vi "MultiModuleAssembly.vi"() -> ()   [LabVIEW 2019]
panel:
  in  "GoHome":bool
  out "Error Out":errorcluster
  in  "Error In":errorcluster
  out "CurrentGlueCommand":string
  in  "GlPatternPCB2":path=path "C:/Users/TTUHEP/Documents/LabVIEW/Data/Patterns/NSH_10-28-2021_rotated1_Minus120degrees_edgesModified_circlesFirst_Combined_version2.ngc"
  in  "Position2":bool=TRUE
  in  "Position1":bool=TRUE
  in  "Glue2":bool=TRUE
  in  "Glue1":bool=TRUE
  in  "Operations2":T1={"GoToToolPos"=TRUE, "PickTool"=TRUE, "GoToSenPCB"=TRUE, "PickSiPCB"=TRUE, "GoToBP"=TRUE, "DropTool"=TRUE}
  in  "Zone":enum16{"ZoneA", "ZoneB", "ZoneC", "ZoneD"}(ring)
  in  "AssmbType":enum16{"Sensor", "PCB"}(ring)=enum."PCB"
  in  "Operations1":T1={"GoToToolPos"=TRUE, "PickTool"=TRUE, "GoToSenPCB"=TRUE, "PickSiPCB"=TRUE, "GoToBP"=TRUE, "DropTool"=TRUE}
  in  "PressureSiPCB2":dbl[](array[numeric])=[15.0, 14.0, 8.0, 0.0]
  in  "PressureBPSi2":dbl[](array[numeric])=[30.0, 30.0, 15.0, 0.0]
  in  "SyringePosition2":T2={"SyringeX"=385.441, "SyringeY"=892.714, "SyringeZ"=75.0} {"SyringeX" format="%#_13g"; "SyringeY" format="%#_13g"}
  in  "SyringePosition1":T2={"SyringeX"=333.933, "SyringeY"=1082.586, "SyringeZ"=74.0} {"SyringeX" format="%#_13g"; "SyringeY" format="%#_13g"}
  in  "PressureSiPCB1":dbl[](array[numeric])=[15.0, 14.0, 8.0, 0.0]
  in  "PressureBPSi1":dbl[](array[numeric])=[30.0, 30.0, 15.0, 0.0]
  in  "GlueVISA":refnum<visa-resource-name>="COM5"
  in  "GlPatternSi":path=path "C:/Users/TTUHEP/Documents/LabVIEW/Data/Patterns/Final_Patern/PCB_base_10-25-2021_3layers_Combined_Final.ngc"
  in  "GlPatternPCB1":path=path "C:/Users/TTUHEP/Documents/LabVIEW/Data/Patterns/NSH_10-28-2021_rotated1_Minus120degrees_edgesModified_circlesFirst_Combined_version2.ngc"
  in  "SyringeToPlateGap(um)":string="330"
  in  "Initialize":T3
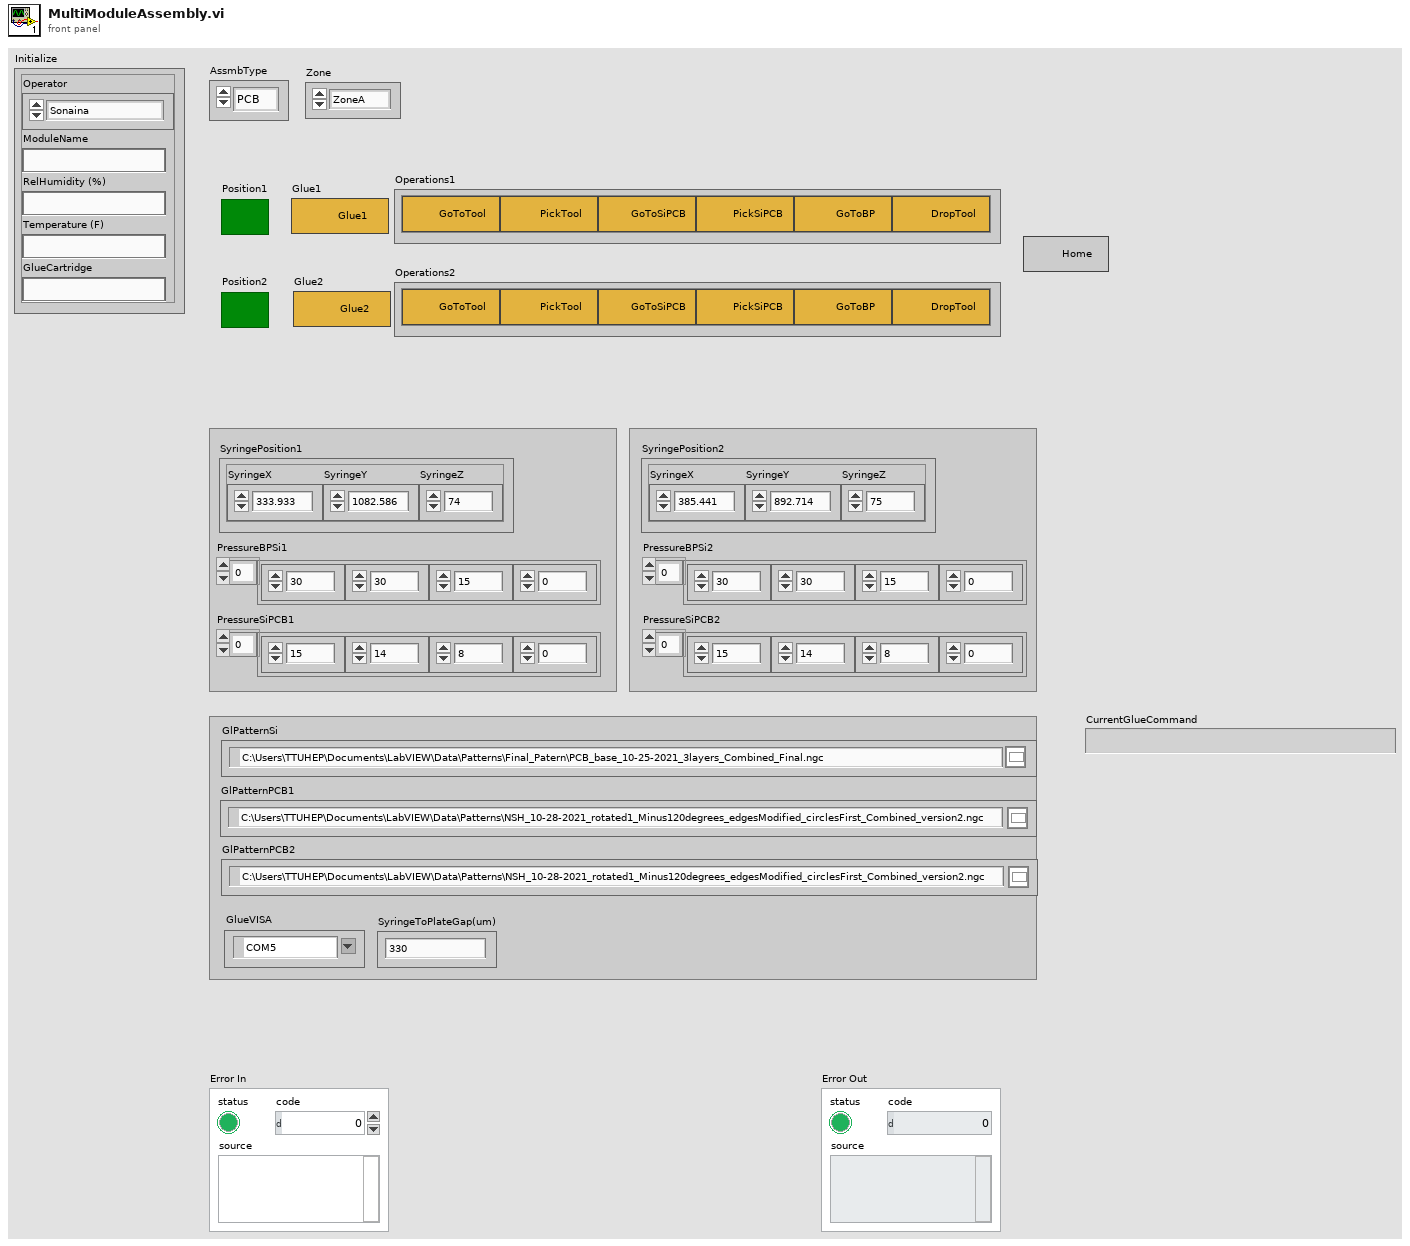
[diagram p1: front panel]
types:
  T1 = cluster{"GoToToolPos":bool, "PickTool":bool, "GoToSenPCB":bool, "PickSiPCB":bool, "GoToBP":bool, "DropTool":bool}
  T2 = cluster{"SyringeX":dbl, "SyringeY":dbl, "SyringeZ":dbl}
  T3 = cluster{"Operator":enum16{"Sonaina", "Vladimir", "Vinay", "Other"}, "ModuleName":string, "RelHumidity (%)":string, "Temperature (F)":string, "GlueCartridge":string}
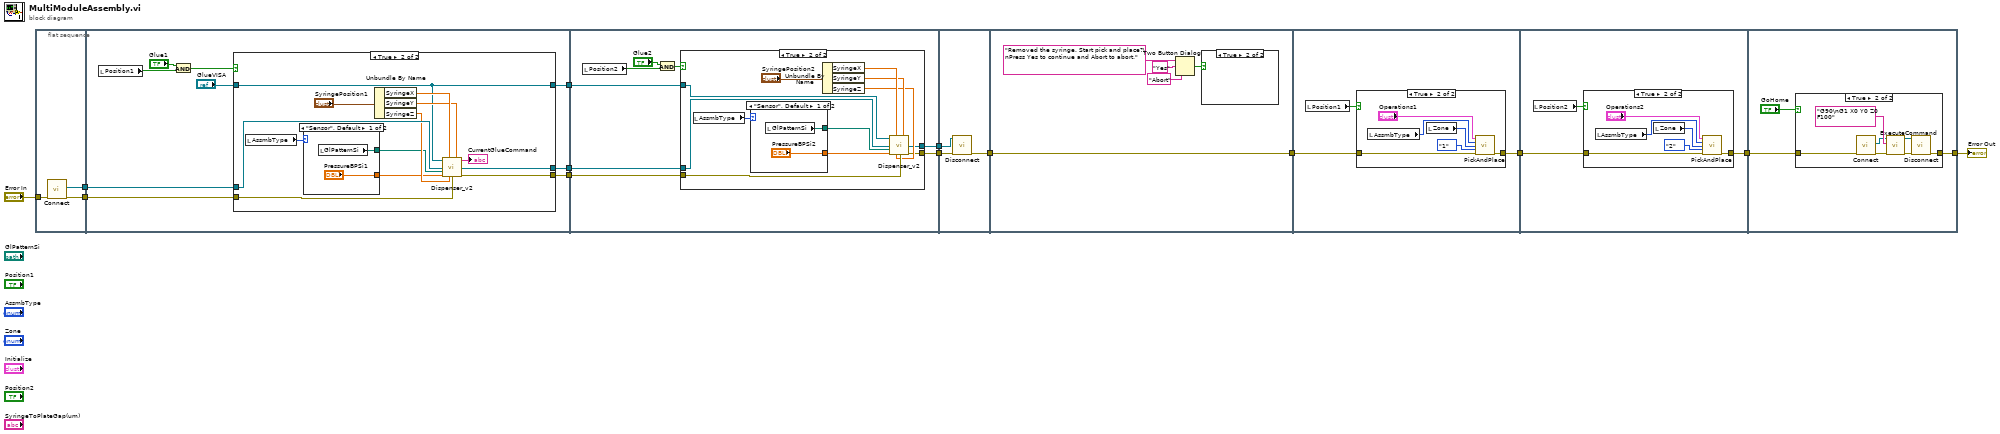
[diagram p0: block diagram]
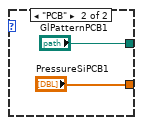
[diagram p3: hidden frame]
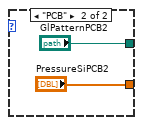
[diagram p5: hidden frame]
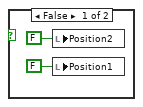
[diagram p6: hidden frame]
diagram:
  n1 = flat-sequence {
    tunnel: [w16] -> w13
    tunnel: [w15] -> w12
    tunnel: "Error In" -> [w14]
    tunnel: w13 -> [w25]
    tunnel: w12 -> [w24]
    tunnel: [w20] -> w11
    tunnel: [w19] -> w10
    tunnel: [w17] -> w7
    tunnel: w11 -> [w50]
    tunnel: w10 -> [w49]
    tunnel: [w48] -> w9
    tunnel: [w47] -> w8
    tunnel: w7 -> [w46]
    tunnel: w9 -> [w74]
    tunnel: w8 -> [w73]
    tunnel: [w72] -> w2
    tunnel: w2 -> [w79]
    tunnel: [w79] -> w1
    tunnel: w1 -> [w84]
    tunnel: [w82] -> w6
    tunnel: w6 -> [w93]
    tunnel: [w92] -> w3
    tunnel: [w103] -> w4
    tunnel: w3 -> [w102]
    frame #0 {
      n2 = call "Connect.vi"("error in (no error)"=w14) -> ("error out"=w15:errorcluster, "controller"=w16:refnum<k24>)  [unwired: 9 in]
    }
    frame #1 {
      n3 = local read "Position1"() -> (w22:bool)
      n4 = And(x="Glue1", y=w22) -> (x .and. y?=w21:bool)
      n5 = case shown="True" w21 {
        tunnel: w25 -> [w28 w41]
        tunnel: w24 -> [w27 w40]
        tunnel: [w28 w34] -> w20
        tunnel: [w27 w33] -> w19
        tunnel: "GlueVISA" -> [w26 w29]
        tunnel: [w26 w29] -> w17
        frame False {
        }
        frame True {
          n6 = local read "AssmbType"() -> (w32:enum16{"Sensor", "PCB"})
          n7 = case shown="\"Sensor\", Default" w32 {
            tunnel: [w43 "GlPatternPCB1"] -> w31
            tunnel: ["PressureBPSi1" "PressureSiPCB1"] -> w30
            frame "Sensor", Default {
              n8 = local read "GlPatternSi"() -> (w43:path)
            }
            frame "PCB" {
            }
          }
          n9 = Unbundle By Name("SyringePosition1") -> ("SyringeX"=w38:dbl, "SyringeY"=w37:dbl, "SyringeZ"=w36:dbl)
          n10 = call "Dispenser_v2.vi"("VISA resource name"=w29, "X"=w38, "Y"=w37, "controller in"=w41, "Path"=w31, "Pressure"=w30, "Z"=w36, "error in (no error)"=w40) -> ("Comm"=→"CurrentGlueCommand":string, "controller out"=w34:refnum<k24>, "error out"=w33:errorcluster)  [unwired: 3 in, 2 out]
        }
      }
    }
    frame #2 {
      n11 = local read "Position2"() -> (w52:bool)
      n12 = And(x="Glue2", y=w52) -> (x .and. y?=w51:bool)
      n13 = case shown="True" w51 {
        tunnel: w50 -> [w55 w67]
        tunnel: w49 -> [w54 w66]
        tunnel: [w55 w61] -> w48
        tunnel: [w54 w60] -> w47
        tunnel: w46 -> [_ w59]
        frame False {
        }
        frame True {
          n14 = local read "AssmbType"() -> (w56:enum16{"Sensor", "PCB"})
          n15 = case shown="\"Sensor\", Default" w56 {
            tunnel: ["PressureBPSi2" "PressureSiPCB2"] -> w58
            tunnel: [w69 "GlPatternPCB2"] -> w57
            frame "Sensor", Default {
              n16 = local read "GlPatternSi"() -> (w69:path)
            }
            frame "PCB" {
            }
          }
          n17 = Unbundle By Name("SyringePosition2") -> ("SyringeX"=w64:dbl, "SyringeY"=w63:dbl, "SyringeZ"=w62:dbl)
          n18 = call "Dispenser_v2.vi"("VISA resource name"=w59, "X"=w64, "Y"=w63, "controller in"=w67, "Path"=w57, "Pressure"=w58, "Z"=w62, "error in (no error)"=w66) -> ("controller out"=w61:refnum<k24>, "error out"=w60:errorcluster)  [unwired: 3 in, 3 out]
        }
      }
    }
    frame #3 {
      n19 = call "Disconnect.vi"("error in (no error)"=w73, "controller"=w74) -> ("error out"=w72:errorcluster)  [unwired: 9 in]
    }
    frame #4 {
      n20 = Two Button Dialog(message="Removed the syringe. Start pick and place?\nPress Yes to continue and Abort to abort.", 1:"Abort" ("F button name (\"Cancel\")"), 2:"Yes" ("button name (\"OK\")")) -> (T button?=w76:bool)
      n21 = case shown="True" w76 {
        frame False {
          n22 = local write "Position2"(FALSE ("Position2")) -> ()
          n23 = local write "Position1"(FALSE ("Position1")) -> ()
        }
        frame True {
        }
      }
    }
    frame #5 {
      n24 = local read "Position1"() -> (w83:bool)
      n25 = case shown="True" w83 {
        tunnel: w84 -> [w85 w89]
        tunnel: [w85 w86] -> w82
        frame False {
        }
        frame True {
          n26 = local read "AssmbType"() -> (w88:enum16{"Sensor", "PCB"})
          n27 = local read "Zone"() -> (w87:enum16{"ZoneA", "ZoneB", "ZoneC", "ZoneD"})
          n28 = call "PickAndPlace.vi"("Operations"="Operations1", "AssmbType"=w88, "Zone"=w87, "Position"=enum16{"1", "2"}."1", "Error In"=w89) -> ("Error Out"=w86:errorcluster)  [unwired: 10 in]
        }
      }
    }
    frame #6 {
      n29 = local read "Position2"() -> (w94:bool)
      n30 = case shown="True" w94 {
        tunnel: w93 -> [w95 w97]
        tunnel: [w95 w96] -> w92
        frame False {
        }
        frame True {
          n31 = local read "AssmbType"() -> (w100:enum16{"Sensor", "PCB"})
          n32 = local read "Zone"() -> (w101:enum16{"ZoneA", "ZoneB", "ZoneC", "ZoneD"})
          n33 = call "PickAndPlace.vi"("Operations"="Operations2", "AssmbType"=w100, "Zone"=w101, "Position"=enum16{"1", "2"}."2", "Error In"=w97) -> ("Error Out"=w96:errorcluster)  [unwired: 10 in]
        }
      }
    }
    frame #7 {
      n34 = case shown="True" "GoHome" {
        tunnel: [w105 w106] -> w103
        tunnel: w102 -> [w105 w107]
        frame False {
        }
        frame True {
          n35 = call "Connect.vi"("error in (no error)"=w107) -> ("error out"=w112:errorcluster, "controller"=w109:refnum<k24>)  [unwired: 9 in]
          n36 = call "ExecuteCommand.vi"("error in (no error)"=w112, "Command Code"="G90\nG1 X0 Y0 Z0 F100", "controller in"=w109) -> ("error out"=w111:errorcluster, "controller out"=w108:refnum<k24>)  [unwired: 6 in, 1 out]
          n37 = call "Disconnect.vi"("error in (no error)"=w111, "controller"=w108) -> ("error out"=w106:errorcluster)  [unwired: 9 in]
        }
      }
    }
  }
  "Error Out" <- w4
